vi "Initialize.vi"(6 "timeout in ms":i32=2000, 7 "Engine Configuration":refnum<class "engine configuration.lvclass">, 8 "error in":errorcluster, 9 "Module Configurations":refnum<class "TBM module configuration.lvclass">[](array[class]), 10 "Modules":refnum<class "TBM module execution interface.lvclass">[](array[class]), 11 "Standard Engine in":refnum<class "synchronous engine runtime.lvclass">) -> (0 "error out":errorcluster, 3 "Standard Engine out":refnum<class "synchronous engine runtime.lvclass">)   [LabVIEW 2013, in "synchronous engine runtime.lvclass"]
uses:
  synchronous engine runtime.lvclass
  Configuration/synchronous engine configuration.lvclass
  <vilib>/NI/Tag Bus Module Framework/module configuration/TBM module configuration.lvclass
  <vilib>/NI/Tag Bus Module Framework/runtime/TBM module execution interface.lvclass
  Engine Configuration/engine configuration.lvclass
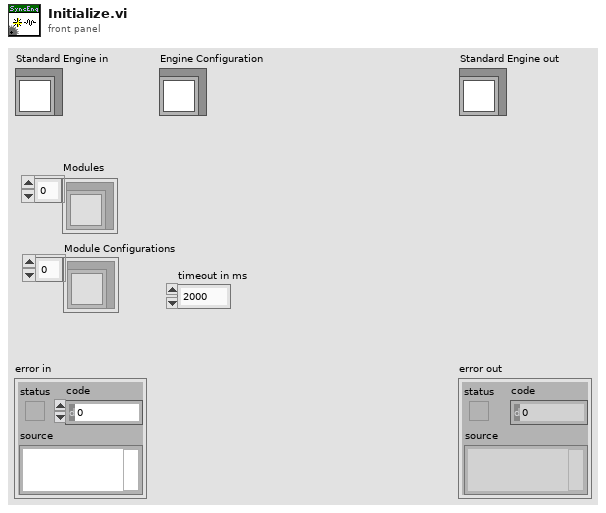
[diagram p1: front panel]
types:
  T1 = typedef "synchronous engine runtime.lvclass/Engine Data.ctl" = cluster{"Main Tag Data":T2, "Module Info":T3, "Safe State?":bool, "engine timing source":refnum<class "TBM timing source.lvclass">, "Timing Source dt":u32, "Processor":i32, "Priority":i32}
  T2 = typedef "tag bus.lvlib/data table.lvlib/data table.ctl" = cluster{"Double":dbl[], "Single":sgl[], "I64":i64[], "I32":i32[], "I16":i16[], "I8":i8[], "U64":u64[], "U32":u32[], "U16":u16[], "U8":u8[], "Boolean":bool[], "String":string[], "Array of Double":cluster{"DBL Array":dbl[]}[], "Array of Single":cluster{"SGL Array":sgl[]}[], "Array of I64":cluster{"I64 Array":i64[]}[], "Array of I32":cluster{"I32 Array":i32[]}[], "Array of I16":cluster{"I16 Array":i16[]}[], "Array of I8":cluster{"I8 Array":i8[]}[], "Array of U64":cluster{"U64 Array":u64[]}[], "Array of U32":cluster{"U32 Array":u32[]}[], "Array of U16":cluster{"U16 Array":u16[]}[], "Array of U8":cluster{"U8 Array":u8[]}[], "Array of Boolean":cluster{"Boolean Array":bool[]}[], "Array of String":cluster{"String Array":string[]}[]}
  T3 = typedef "synchronous engine runtime.lvclass/Module Execution Info.ctl" = cluster{"Tag Bus Modules":refnum<class "TBM module execution interface.lvclass">[], "Execute?":bool[], "Input Method Indices":i32[], "Process Method Indices":i32[], "Output Method Indices":i32[], "Input Transfer Specifications":T4[], "Parameter Transfer Specifications":T4[], "Result Transfer Specifications":T4[], "Output Transfer Specifications":T4[], "Module Errors":errorcluster[]}
  T4 = typedef "synchronous engine runtime.lvclass/Data Table with Transfer Spec.ctl" = cluster{"Data Table":T2, "Transfer Specification":T5[]}
  T5 = typedef "tag bus.lvlib/data table.lvlib/transfer specification.ctl" = cluster{"data type":T6, "sink indices":i32[], "source indices":i32[]}
  T6 = typedef "tag bus.lvlib/tag descriptor.lvclass/Data Type.ctl" = enum16{"Double", "Single", "I64", "I32", "I16", "I8", "U64", "U32", "U16", "U8", "Boolean", "String", "Array of Double", "Array of Single", "Array of I64", "Array of I32", "Array of I16", "Array of I8", "Array of U64", "Array of U32", "Array of U16", "Array of U8", "Array of Boolean", "Array of String"}
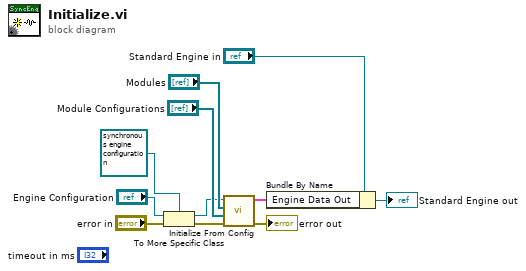
[diagram p0: block diagram]
diagram:
  n1 = To More Specific Class(target class=refnum<class "synchronous engine configuration.lvclass"> refnum ("Engine Configuration"), reference="Engine Configuration", error in="error in") -> (specific class reference=w1:refnum<class "synchronous engine configuration.lvclass">, error out=w6:errorcluster)
  n2 = call "Initialize From Config.vi"("error in"=w6, "Module Configurations"="Module Configurations", "Modules"="Modules", "Engine Configuration"=w1) -> ("error out"=→"error out":errorcluster, "Engine Data Out"=w2:T1)  [unwired: 6 in]
  n3 = Bundle By Name(cluster="Standard Engine in", "Engine Data Out"=w2) -> (→"Standard Engine out":refnum<class "synchronous engine runtime.lvclass">)
